vi "Get Water Level.vi"(8 "error in (no error)":cluster{"状态":bool, "代码":i32, "源":string} caption="错误输入（无错误）", 11 "硬件水位输入":refnum<class "HW Water Level.lvclass">) -> (0 "error out":cluster{"状态":bool, "代码":i32, "源":string} caption="错误输出", 2 "水位":dbl)   [LabVIEW 2013, in "HW Water Level.lvclass"]
uses:
  HW Water Level.lvclass
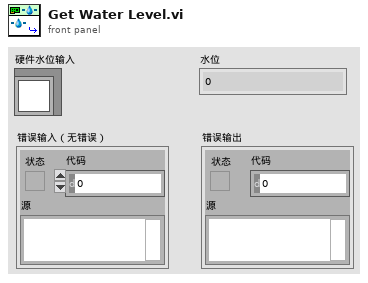
[diagram p1: front panel]
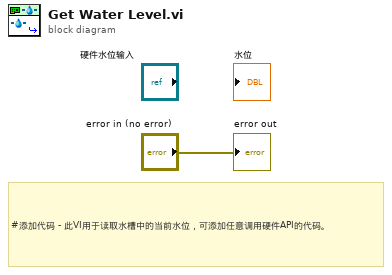
[diagram p0: block diagram]
diagram:
  # "#添加代码 - 此VI用于读取水槽中的当前水位，可添加任意调用硬件API的代码。"
  "error out" <- "error in (no error)"
